vi "Demo_GetSoundFromMovie.vi"() -> ()   [LabVIEW 2024]
doc: "Extract the samples of the first sound track of the movie. \nSupport all QuickTime formats (MOV, WAV, mp4, AAC, µLaw, etc.)\n\n© Chris Salzmann 1994 - 2003"
uses:
  <userlib>/ImageProcessing/QTLIB_2595_LV86/QT_File.ctl
  <userlib>/ImageProcessing/QTLIB_2595_LV86/QT_Sound.ctl
panel:
  in  "Play Sound":bool
  out "Sound duration [s]":dbl=9.34
  in  "from [s]":dbl
  out "Sound":i16[][](graph)
  out "Sound out":T1 {"Rate" format="%x"}
  out "error out":errorcluster={"status"=TRUE, "code"=-2015, "source"="GetSound()"}
  in  "duration (0: all) [s]":dbl=1.0
  in  "Sound file path":path=path "/BootX/Users/chris/Desktop/Sound.mov"
  # "© Chris Salzmann - 2003"
  # "Extract the samples of the first sound track of the movie. \nSupport all QuickTime formats (MOV, WAV, mp4, AAC, µLaw, etc.)\n\n © Chris Salzmann 1994 - 2005"
  # "Extract"
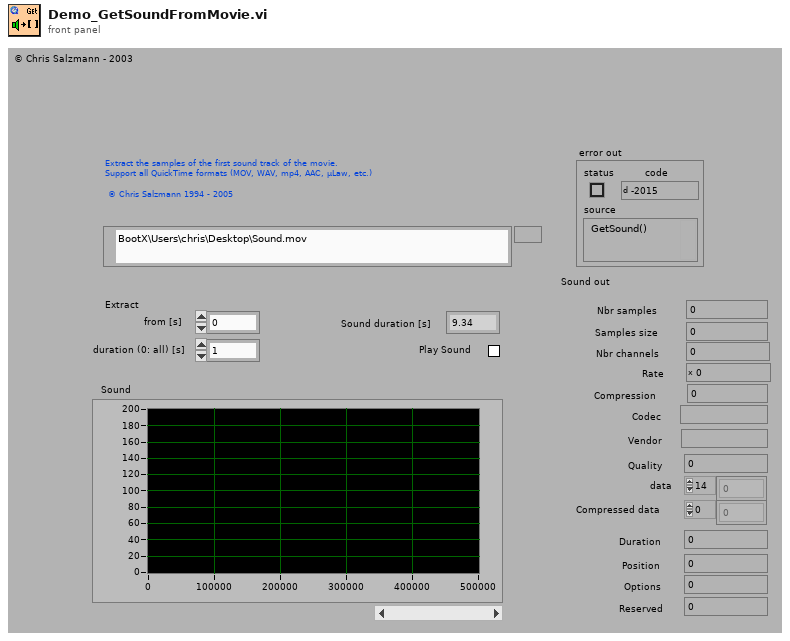
[diagram p1: front panel]
types:
  T1 = typedef "QT_Sound.ctl" = cluster{"Nbr samples":i32, "Samples size":i32, "Nbr channels":i32, "Rate ":i32, "Compression":i32, "Codec":string, "Vendor":string, "Quality":i32, "data":i16[], "Compressed data":u8[], "Duration":i32, "Position":i32, "Options":i32, "Reserved":i32}
  T2 = typedef "QT_File.ctl" = cluster{"Paths":string[], "Options":i32, "Dialogs":u32, "Reserved":i32}
  T3 = typedef "QT_Ref.ctl" = refnum<k1>
  T4 = typedef "QT_MovieInfo.ctl" = cluster{"Author":string, "Info":string, "Copyright":string, "Time scale":i32, "Duration":i32, "Width":i32, "Height":i32, "Nbr Tracks":i32, "Tracks":T5[], "Reserved":i32, "Reserved 2":i32}
  T5 = typedef "QT_Track.ctl" = cluster{"Type":i32, "Samples":i32, "Size":i32, "Compression":i32, "Codec":string, "Vendor":string, "Quality":i32, "Temporal":i32, "Rate ":dbl, "ticks/sec":i32, "Options":i32, "Reserved":i32}
  T6 = typedef "Sound Format.ctl" = cluster{"sound quality":enum16{"mono", "stereo"}, "rate":enum16{"11025", "22050", "44100", "8000"}, "bits per sample":enum16{"8 bit", "16 bit"}}
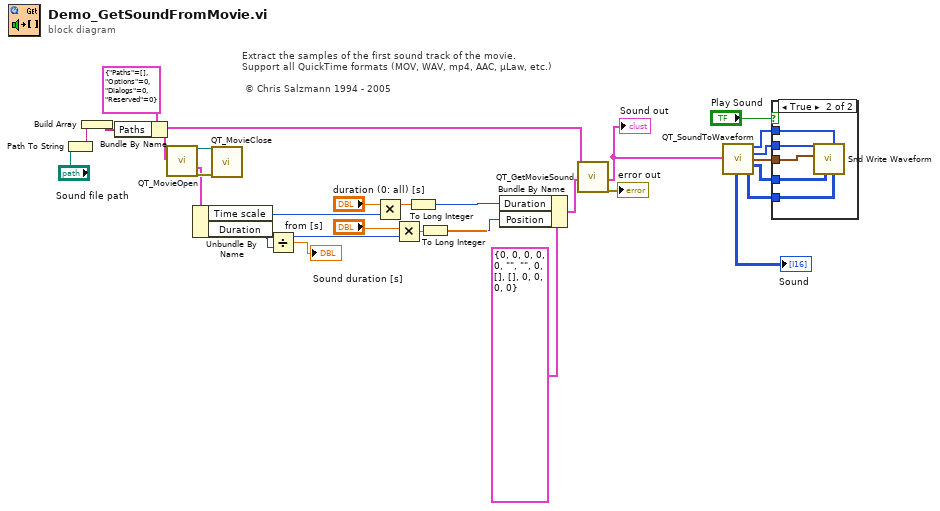
[diagram p0: block diagram]
diagram:
  # "Extract the samples of the first sound track of the movie. \nSupport all QuickTime formats (MOV, WAV, mp4, AAC, µLaw, etc.)\n\n © Chris Salzmann 1994 - 2005"
  n1 = Path To String(path="Sound file path") -> (string=w27:string)
  n2 = Build Array(w27) -> (w23:string[])
  n3 = Bundle By Name(cluster=T2 {"Paths"=[], "Options"=0, "Dialogs"=0, "Reserved"=0} ("File Settings"), "Paths"=w23) -> (w21:T2)
  n4 = call <userlib>:"QT_MovieOpen.vi"("File Settings"=w21) -> ("QT Ref Out"=w20:T3, "Movie info"=w18:T4, "error out"=w19:errorcluster)  [unwired: 2 in, 14 out]
  n5 = Unbundle By Name(w18) -> ("Time scale"=w10:i32, "Duration"=w11:i32)
  n6 = call <userlib>:"QT_MovieClose.vi"("QT Ref In"=w20, "error in (no error)"=w19) -> ()  [unwired: 1 in, 17 out]
  n7 = Divide(x=w11, y=w10) -> (x/y=→"Sound duration [s]":dbl)
  n8 = Multiply(x="duration (0: all) [s]", y=w10) -> (x*y=w16:dbl)
  n9 = Multiply(x="from [s]", y=w10) -> (x*y=w14:dbl)
  n10 = To Long Integer(number=w16) -> (32bit integer=w12:i32)
  n11 = To Long Integer(number=w14) -> (32bit integer=w13:i32)
  n12 = Bundle By Name(cluster=T1 {"Nbr samples"=0, "Samples size"=0, "Nbr channels"=0, "Rate "=0, "Compression"=0, "Codec"="", "Vendor"="", "Quality"=0, "data"=[], "Compressed data"=[], "Duration"=0, "Position"=0, "Options"=0, "Reserved"=0} ("Sound in"), "Duration"=w12, "Position"=w13) -> (w22:T1)
  n13 = call <userlib>:"QT_GetMovieSound.vi"("File Settings"=w21, "Sound in"=w22) -> ("Sound out"=w8:T1, "error out"=→"error out":errorcluster)  [unwired: 3 in, 13 out]
  "Sound out" <- w8
  n14 = call <userlib>:"QT_SoundToWaveform.vi"("Sound in"=w8) -> ("mono 16-bit"=w5:i16[], "mono 8-bit"=w4:u8[], "sound format"=w6:T6, "stereo 8-bit"=w2:u8[][], "display"=→"Sound":i16[][], "stereo 16-bit"=w7:i16[][])  [unwired: 9 out]
  n15 = case shown="True" "Play Sound" {
    tunnel: w4 -> [_ w33]
    tunnel: w5 -> [_ w32]
    tunnel: w2 -> [_ w31]
    tunnel: w7 -> [_ w30]
    tunnel: w6 -> [_ w29]
    frame False {
    }
    frame True {
      n16 = call <vilib>:"Snd Write Waveform.vi"("stereo 16-bit"=w30, "mono 16-bit"=w32, "stereo 8-bit"=w31, "mono 8-bit"=w33, "sound format"=w29) -> ()  [unwired: 2 in, 5 out]
    }
  }
